vi "Write Image Date.vi"(8 "error in (no error)":errorcluster, 10 "SYSTEMTIME":T1, 11 "Simulated_CCD_Camera in":refnum<class "Simulated_CCD_Camera.lvclass">) -> (0 "error out":errorcluster, 3 "Simulated_CCD_Camera out":refnum<class "Simulated_CCD_Camera.lvclass">)   [LabVIEW 2018, in "Simulated_CCD_Camera.lvclass"]
uses:
  Simulated_CCD_Camera.lvclass
  <userlib>/atmcd32d.llb/SYSTEMTIME structure typedef.ctl
  Simulated_CCD_Camera.lvclass/Simulated_CCD_Camera.ctl
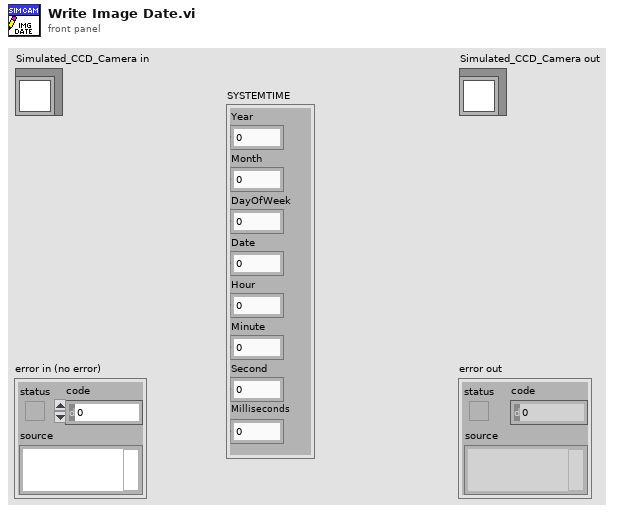
[diagram p1: front panel]
types:
  T1 = typedef "SYSTEMTIME structure typedef.ctl" = cluster{"Year":u16, "Month":u16, "DayOfWeek":u16, "Date":u16, "Hour":u16, "Minute":u16, "Second":u16, "Milliseconds":u16}
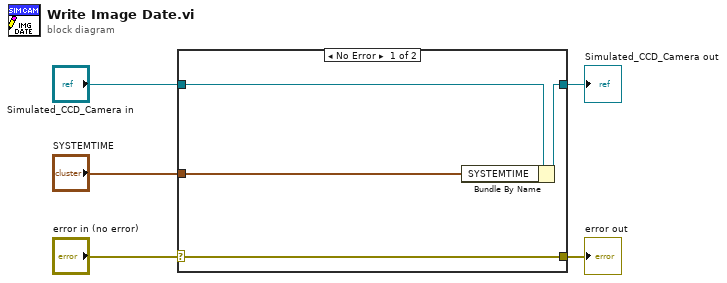
[diagram p0: block diagram]
diagram:
  n1 = case shown="No Error" "error in (no error)" {
    selector: "error in (no error)" -> [w9 w10]
    tunnel: [w9 w10] -> w4
    tunnel: [w7 w11] -> w2
    tunnel: "Simulated_CCD_Camera in" -> [w8 w11]
    tunnel: "SYSTEMTIME" -> [w6 _]
    frame No Error {
      n2 = Bundle By Name(cluster=w8, "SYSTEMTIME"=w6) -> (w7:refnum<class "Simulated_CCD_Camera.lvclass">)
    }
    frame Error {
    }
  }
  "error out" <- w4
  "Simulated_CCD_Camera out" <- w2
